vi "Motors Position Save.vi"(4 "file path":path=path "C:/LabView VIs/IPES SubVIs/saved_positions.txt", 5 "error in":errorcluster, 6 "Position Name":string, 7 "Theta (deg)":dbl, 8 "Z (mm)":dbl, 9 "Y (mm)":dbl, 10 "X (mm)":dbl) -> (0 "error out":errorcluster)   [LabVIEW 2018]
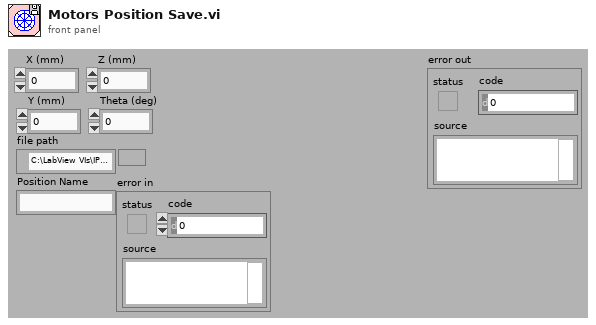
[diagram p1: front panel]
types:
  T1 = enum16{"open", "replace", "create", "open or create", "replace or create", "replace or create with confirmation"}
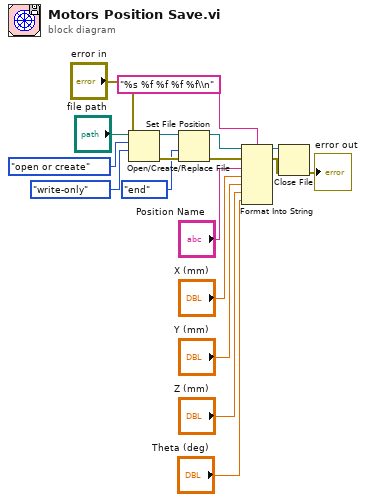
[diagram p0: block diagram]
diagram:
  n1 = Open/Create/Replace File(file path (use dialog)="file path", error in="error in", operation (0:open)=T1."open or create", access (0:read/write)=enum16{"read/write", "read-only", "write-only"}."write-only") -> (refnum out=w4:refnum<file>, error out=w6:errorcluster)  [unwired: 2 in, 1 out]
  n2 = Set File Position(refnum=w4, from (0:start)=enum16{"start", "end", "current"}."end", error in=w6) -> (refnum out=w3:refnum<file>, error out=w5:errorcluster)  [unwired: 1 in]
  n3 = Format Into String(format string="%s %f %f %f %f\\n", initial string=w3, error in=w5, "Position Name", "X (mm)", "Y (mm)", "Z (mm)", "Theta (deg)") -> (resulting string=w9:refnum<file>, error out=w8:errorcluster)
  n4 = Close File(refnum=w9, error in=w8) -> (error out=→"error out":errorcluster)  [unwired: 1 out]
